vi "Serial_read_err_check.vi"(7 "timeout":u32, 8 "error in (no error)":errorcluster, 9 "dt":u32, 11 "read buffer":string) -> (3 "error?":bool)   [LabVIEW 2017]
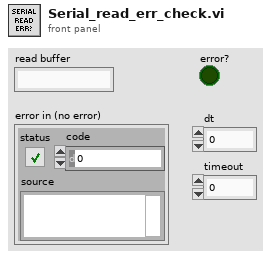
[diagram p1: front panel]
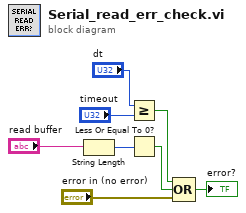
[diagram p0: block diagram]
diagram:
  n1 = String Length(string="read buffer") -> (length=w5:i32)
  n2 = Greater Or Equal?(x="dt", y="timeout") -> (x >= y?=w1:bool)
  n3 = Less Or Equal To 0?(x=w5) -> (x <= 0?=w6:bool)
  n4 = Compound Arithmetic op=OR(w1, w6, "error in (no error)") -> (→"error?":bool)
